vi "pwm przod jazda.vi"(9 "max pwm przod":i32, 10 "Y axis":i32) -> (3 "Numeric":i32)   [LabVIEW 2015]
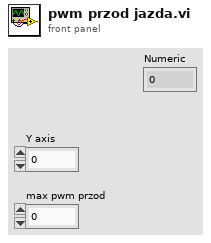
[diagram p1: front panel]
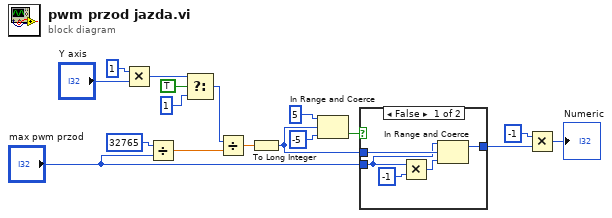
[diagram p0: block diagram]
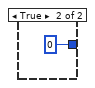
[diagram p2: hidden frame]
diagram:
  n1 = Multiply(x=1, y="Y axis") -> (x*y=w8:i32)
  n2 = Divide(x=32765 ("y"), y="max pwm przod") -> (x/y=w13:dbl)
  n3 = Select(t=w8, s=TRUE, f=1) -> (s? t:f=w3:i32)
  n4 = Divide(x=w3, y=w13) -> (x/y=w5:dbl)
  n5 = To Long Integer(number=w5) -> (32bit integer=w12:i32)
  n6 = In Range and Coerce(upper limit=5 ("y"), x=w12, lower limit=-5 ("y")) -> (In Range?=w2:bool)  [unwired: 1 out]
  n7 = case shown="False" w2 {
    tunnel: [w22 0 ("y")] -> w11
    tunnel: w12 -> [w21 _]
    tunnel: "max pwm przod" -> [w18 _]
    frame False {
      n8 = Multiply(x=w18, y=-1) -> (x*y=w20:i32)
      n9 = In Range and Coerce(upper limit=w18, x=w21, lower limit=w20) -> (coerced(x)=w22:i32)  [unwired: 1 out]
    }
    frame True {
    }
  }
  n10 = Multiply(x=-1, y=w11) -> (x*y=→"Numeric":i32)
